vi "Main.vi"() -> ()   [LabVIEW 2021]
uses:
  TypeDef/StateMachine.ctl
  TypeDef/KeyDown.ctl
  GlobalVariables/Global_KeyDown.vi
  GlobalVariables/Board_Colors.vi
panel:
  in  "stop":bool
  out "Scoreboard":i32
  out "Level":u32[][](array[colorbox])
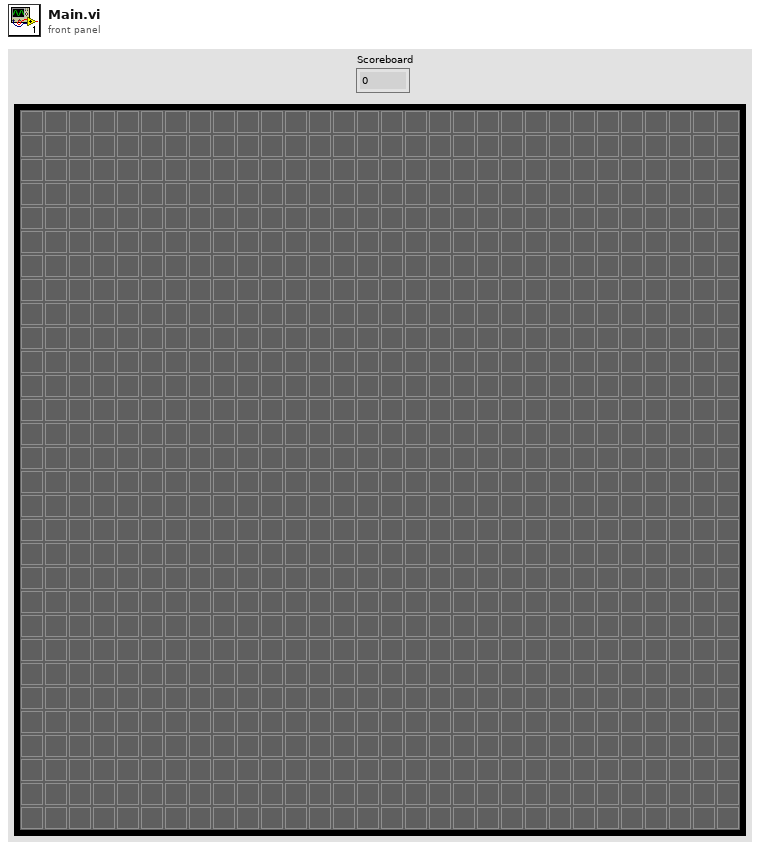
[diagram p1: front panel]
types:
  T1 = typedef "KeyDown.ctl" = enum16{"Up", "Down", "Left", "Right"}
  T2 = typedef "StateMachine.ctl" = enum16{"Init", "Game Logic", "Snake Growth", "Move", "Wait", "Food", "Update", "Game over"}
  T3 = typedef "eventvkey.ctl" = enum16{"ASCII", "Enter", "Return", "Shift", "Ctrl", "Alt", "Cmd", "Opt", "Caps", "NumLock", "Clear", "Break", "Up", "Down", "Left", "Right", "Insert", "Delete", "Home", "End", "PageUp", "PageDown", "Escape", "Help", "Pause", "ScrollLock", "F1", "F2", "F3", "F4", "F5", "F6", "F7", "F8", "F9", "F10", "F11", "F12", "F13", "F14", "F15", "F16", "F17", "F18", "F19", "F20", "F21", "F22", "F23", "F24", "Play", "VolumeUp", "VolumeDown", "Mute", "Two Byte Char"}
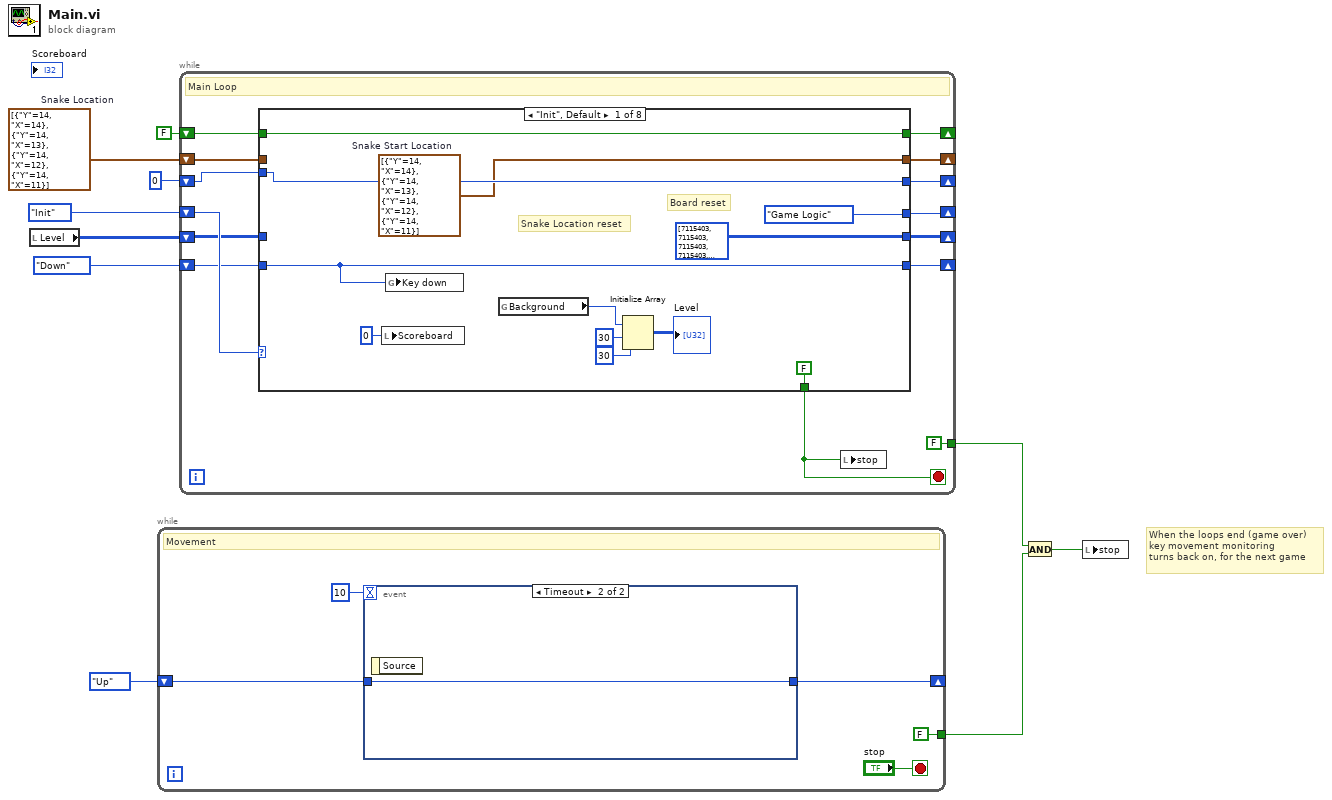
[diagram p0: block diagram]
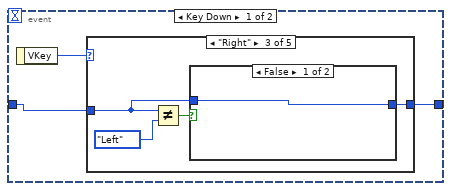
[diagram p2: hidden frame]
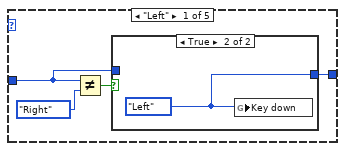
[diagram p3: hidden frame]
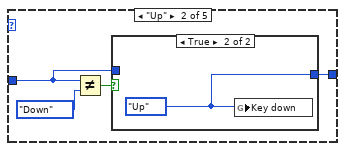
[diagram p5: hidden frame]
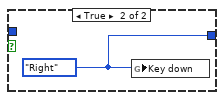
[diagram p7: hidden frame]
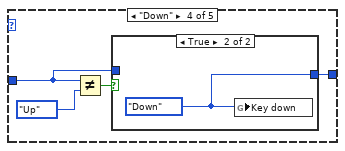
[diagram p8: hidden frame]
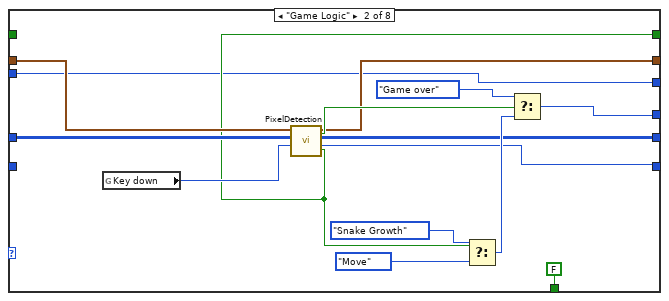
[diagram p11: hidden frame]
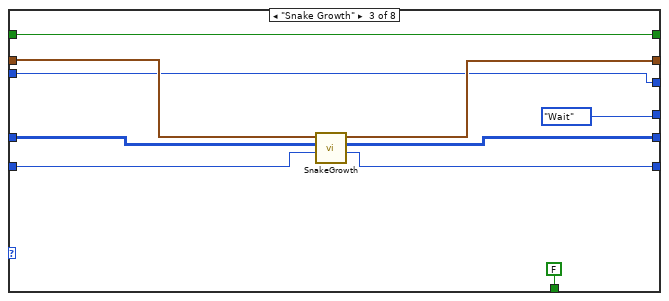
[diagram p12: hidden frame]
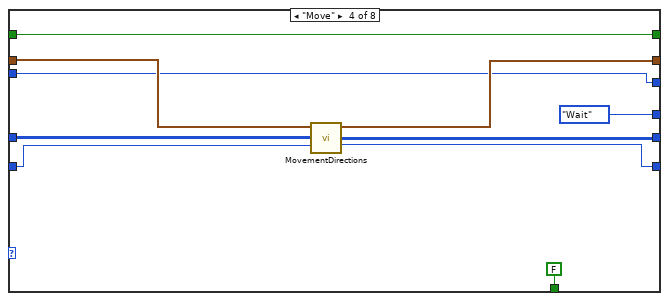
[diagram p13: hidden frame]
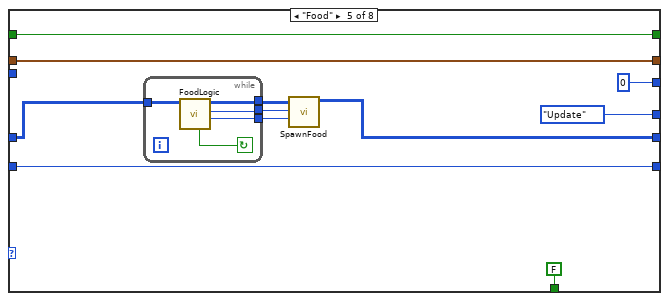
[diagram p14: hidden frame]
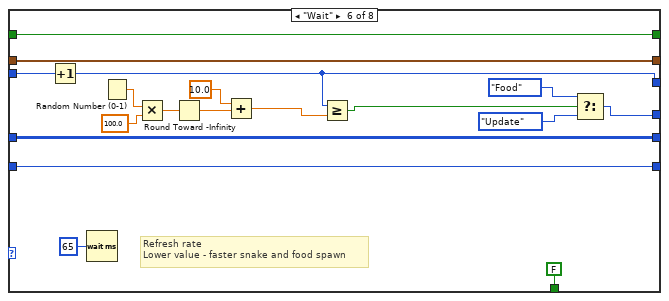
[diagram p15: hidden frame]
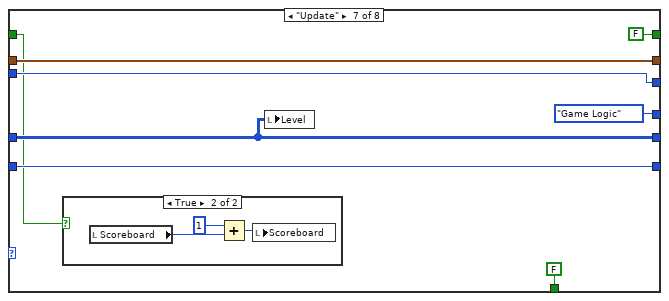
[diagram p16: hidden frame]
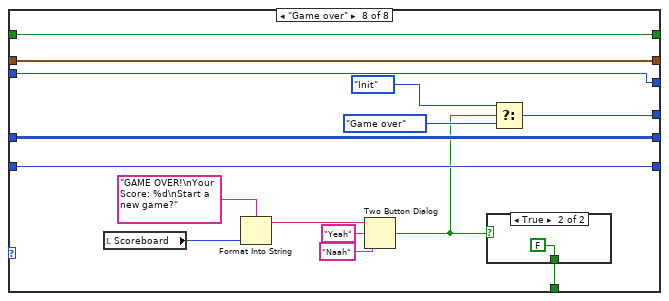
[diagram p18: hidden frame]
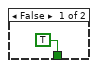
[diagram p19: hidden frame]
diagram:
  w9 = cluster{"Y":i32, "X":i32}[] [{"Y"=14, "X"=14}, {"Y"=14, "X"=13}, {"Y"=14, "X"=12}, {"Y"=14, "X"=11}]  # Snake Location
  # "When the loops end (game over)\nkey movement monitoring\nturns back on, for the next game"
  n1 = local read "Level"() -> (w8:u32[][])
  n2 = while {
    shift-right: [w13] -> _
    shift-left: KeyDown."Up" ("Key down") -> [w14]
    tunnel: [FALSE ("y")] -> w4
    stop <- "stop" stop-if-true
    # "Movement"
    n3 = event shown="[1] Timeout" {
      selector: _ -> [_ _]
      dyn-events: _ -> [_ _]
      timeout: 10 -> [_ _]
      tunnel: [w17 w44] -> w13
      tunnel: w14 -> [w16 w44]
      event Key Down {
        n4 = event-data() -> ("VKey"=w18:T3)  [unwired: 1 in]
        n5 = case shown="\"Right\"" w18 {
          tunnel: [w21 w27 w33 w39 w43] -> w17
          tunnel: w16 -> [w19 w25 w31 w37 w43]
          frame "Left" {
            n6 = Not Equal?(x=w19, y=KeyDown."Right" ("Key down")) -> (x != y?=w22:bool)
            n7 = case shown="True" w22 {
              tunnel: [w23 w24] -> w21
              tunnel: w19 -> [w23 _]
              frame False {
              }
              frame True {
                w24 = KeyDown."Left" ("Key down")
                n8 = global write "Global_KeyDown.vi" "Key down"(w24) -> ()
              }
            }
          }
          frame "Up" {
            n9 = Not Equal?(x=w25, y=KeyDown."Down" ("Key down")) -> (x != y?=w28:bool)
            n10 = case shown="True" w28 {
              tunnel: [w29 w30] -> w27
              tunnel: w25 -> [w29 _]
              frame False {
              }
              frame True {
                w30 = KeyDown."Up" ("Key down")
                n11 = global write "Global_KeyDown.vi" "Key down"(w30) -> ()
              }
            }
          }
          frame "Right" {
            n12 = Not Equal?(x=w31, y=KeyDown."Left" ("Key down")) -> (x != y?=w34:bool)
            n13 = case shown="False" w34 {
              tunnel: [w35 w36] -> w33
              tunnel: w31 -> [w35 _]
              frame False {
              }
              frame True {
                w36 = KeyDown."Right" ("Key down")
                n14 = global write "Global_KeyDown.vi" "Key down"(w36) -> ()
              }
            }
          }
          frame "Down" {
            n15 = Not Equal?(x=w37, y=KeyDown."Up" ("Key down")) -> (x != y?=w40:bool)
            n16 = case shown="True" w40 {
              tunnel: [w41 w42] -> w39
              tunnel: w37 -> [w41 _]
              frame False {
              }
              frame True {
                w42 = KeyDown."Down" ("Key down")
                n17 = global write "Global_KeyDown.vi" "Key down"(w42) -> ()
              }
            }
          }
          frame Default {
          }
        }
      }
      event Timeout {
        n18 = event-data() -> ()  [unwired: 1 in, 1 out]
      }
    }
  }
  n19 = while {
    shift-right: [w53] -> _
    shift-left: StateMachine."Init" -> [w58]
    shift-right: [w56] -> _
    shift-left: KeyDown."Down" ("Key down") -> [w57]
    shift-right: [w55] -> _
    shift-left: w9 -> [w54]
    shift-right: [w52] -> _
    shift-left: w8 -> [w51]
    tunnel: [FALSE] -> w5
    shift-right: [w49] -> _
    shift-left: 0 -> [w48]
    shift-right: [w47] -> _
    shift-left: FALSE -> [w46]
    stop <- w45 stop-if-true
    # "Main Loop"
    n20 = case shown="\"Init\", Default" w58 {
      tunnel: w57 -> [w69 _ w91 w101 w116 w137 w144 w165]
      tunnel: [w69 w79 w90 w100 w116 w137 w144 w165] -> w56
      tunnel: [w60 w77 w94 w104 w114 w139 w147 w164] -> w55
      tunnel: w54 -> [_ w83 w95 w105 w114 w139 w147 w164]
      tunnel: [StateMachine."Game Logic" w74 StateMachine."Wait" StateMachine."Wait" StateMachine."Update" w134 StateMachine."Game Logic" w155] -> w53
      tunnel: [u32[][] [[7115403, 7115403, 7115403, 7115403, 7115403, 7115403, 7115403, 7115403, 7115403, 7115403, 7115403, 7115403, 7115403, 7115403, 7115403, 7115403, 7115403, 7115403, 7115403, 7115403, 7115403, 7115403, 7115403, 7115403, 7115403, 7115403, 7115403, 7115403, 7115403, 7115403], [7115403, 7115403, 7115403, 7115403, 7115403, 7115403, 7115403, 7115403, 7115403, 7115403, 7115403, 7115403, 7115403, 7115403, 7115403, 7115403, 7115403, 7115403, 7115403, 7115403, 7115403, 7115403, 7115403, 7115403, 7115403, 7115403, 7115403, 7115403, 7115403, 7115403], [7115403, 7115403, 7115403, 7115403, 7115403, 7115403, 7115403, 7115403, 7115403, 7115403, 7115403, 7115403, 7115403, 7115403, 7115403, 7115403, 7115403, 7115403, 7115403, 7115403, 7115403, 7115403, 7115403, 7115403, 7115403, 7115403, 7115403, 7115403, 7115403, 7115403], [7115403, 7115403, 7115403, 7115403, 7115403, 7115403, 7115403, 7115403, 7115403, 7115403, 7115403, 7115403, 7115403, 7115403, 7115403, 7115403, 7115403, 7115403, 7115403, 7115403, 7115403, 7115403, 7115403, 7115403, 7115403, 7115403, 7115403, 7115403, 7115403, 7115403], [7115403, 7115403, 7115403, 7115403, 7115403, 7115403, 7115403, 7115403, 7115403, 7115403, 7115403, 7115403, 7115403, 7115403, 7115403, 7115403, 7115403, 7115403, 7115403, 7115403, 7115403, 7115403, 7115403, 7115403, 7115403, 7115403, 7115403, 7115403, 7115403, 7115403], [7115403, 7115403, 7115403, 7115403, 7115403, 7115403, 7115403, 7115403, 7115403, 7115403, 7115403, 7115403, 7115403, 7115403, 7115403, 7115403, 7115403, 7115403, 7115403, 7115403, 7115403, 7115403, 7115403, 7115403, 7115403, 7115403, 7115403, 7115403, 7115403, 7115403], [7115403, 7115403, 7115403, 7115403, 7115403, 7115403, 7115403, 7115403, 7115403, 7115403, 7115403, 7115403, 7115403, 7115403, 7115403, 7115403, 7115403, 7115403, 7115403, 7115403, 7115403, 7115403, 7115403, 7115403, 7115403, 7115403, 7115403, 7115403, 7115403, 7115403], [7115403, 7115403, 7115403, 7115403, 7115403, 7115403, 7115403, 7115403, 7115403, 7115403, 7115403, 7115403, 7115403, 7115403, 7115403, 7115403, 7115403, 7115403, 7115403, 7115403, 7115403, 7115403, 7115403, 7115403, 7115403, 7115403, 7115403, 7115403, 7115403, 7115403], [7115403, 7115403, 7115403, 7115403, 7115403, 7115403, 7115403, 7115403, 7115403, 7115403, 7115403, 7115403, 7115403, 7115403, 7115403, 7115403, 7115403, 7115403, 7115403, 7115403, 7115403, 7115403, 7115403, 7115403, 7115403, 7115403, 7115403, 7115403, 7115403, 7115403], [7115403, 7115403, 7115403, 7115403, 7115403, 7115403, 7115403, 7115403, 7115403, 7115403, 7115403, 7115403, 7115403, 7115403, 7115403, 7115403, 7115403, 7115403, 7115403, 7115403, 7115403, 7115403, 7115403, 7115403, 7115403, 7115403, 7115403, 7115403, 7115403, 7115403], [7115403, 7115403, 7115403, 7115403, 7115403, 7115403, 7115403, 7115403, 7115403, 7115403, 7115403, 7115403, 7115403, 7115403, 7115403, 7115403, 7115403, 7115403, 7115403, 7115403, 7115403, 7115403, 7115403, 7115403, 7115403, 7115403, 7115403, 7115403, 7115403, 7115403], [7115403, 7115403, 7115403, 7115403, 7115403, 7115403, 7115403, 7115403, 7115403, 7115403, 7115403, 7115403, 7115403, 7115403, 7115403, 7115403, 7115403, 7115403, 7115403, 7115403, 7115403, 7115403, 7115403, 7115403, 7115403, 7115403, 7115403, 7115403, 7115403, 7115403], [7115403, 7115403, 7115403, 7115403, 7115403, 7115403, 7115403, 7115403, 7115403, 7115403, 7115403, 7115403, 7115403, 7115403, 7115403, 7115403, 7115403, 7115403, 7115403, 7115403, 7115403, 7115403, 7115403, 7115403, 7115403, 7115403, 7115403, 7115403, 7115403, 7115403], [7115403, 7115403, 7115403, 7115403, 7115403, 7115403, 7115403, 7115403, 7115403, 7115403, 7115403, 7115403, 7115403, 7115403, 7115403, 7115403, 7115403, 7115403, 7115403, 7115403, 7115403, 7115403, 7115403, 7115403, 7115403, 7115403, 7115403, 7115403, 7115403, 7115403], [7115403, 7115403, 7115403, 7115403, 7115403, 7115403, 7115403, 7115403, 7115403, 7115403, 7115403, 7115403, 7115403, 7115403, 7115403, 7115403, 7115403, 7115403, 7115403, 7115403, 7115403, 7115403, 7115403, 7115403, 7115403, 7115403, 7115403, 7115403, 7115403, 7115403], [7115403, 7115403, 7115403, 7115403, 7115403, 7115403, 7115403, 7115403, 7115403, 7115403, 7115403, 7115403, 7115403, 7115403, 7115403, 7115403, 7115403, 7115403, 7115403, 7115403, 7115403, 7115403, 7115403, 7115403, 7115403, 7115403, 7115403, 7115403, 7115403, 7115403], [7115403, 7115403, 7115403, 7115403, 7115403, 7115403, 7115403, 7115403, 7115403, 7115403, 7115403, 7115403, 7115403, 7115403, 7115403, 7115403, 7115403, 7115403, 7115403, 7115403, 7115403, 7115403, 7115403, 7115403, 7115403, 7115403, 7115403, 7115403, 7115403, 7115403], [7115403, 7115403, 7115403, 7115403, 7115403, 7115403, 7115403, 7115403, 7115403, 7115403, 7115403, 7115403, 7115403, 7115403, 7115403, 7115403, 7115403, 7115403, 7115403, 7115403, 7115403, 7115403, 7115403, 7115403, 7115403, 7115403, 7115403, 7115403, 7115403, 7115403], [7115403, 7115403, 7115403, 7115403, 7115403, 7115403, 7115403, 7115403, 7115403, 7115403, 7115403, 7115403, 7115403, 7115403, 7115403, 7115403, 7115403, 7115403, 7115403, 7115403, 7115403, 7115403, 7115403, 7115403, 7115403, 7115403, 7115403, 7115403, 7115403, 7115403], [7115403, 7115403, 7115403, 7115403, 7115403, 7115403, 7115403, 7115403, 7115403, 7115403, 7115403, 7115403, 7115403, 7115403, 7115403, 7115403, 7115403, 7115403, 7115403, 7115403, 7115403, 7115403, 7115403, 7115403, 7115403, 7115403, 7115403, 7115403, 7115403, 7115403], [7115403, 7115403, 7115403, 7115403, 7115403, 7115403, 7115403, 7115403, 7115403, 7115403, 7115403, 7115403, 7115403, 7115403, 7115403, 7115403, 7115403, 7115403, 7115403, 7115403, 7115403, 7115403, 7115403, 7115403, 7115403, 7115403, 7115403, 7115403, 7115403, 7115403], [7115403, 7115403, 7115403, 7115403, 7115403, 7115403, 7115403, 7115403, 7115403, 7115403, 7115403, 7115403, 7115403, 7115403, 7115403, 7115403, 7115403, 7115403, 7115403, 7115403, 7115403, 7115403, 7115403, 7115403, 7115403, 7115403, 7115403, 7115403, 7115403, 7115403], [7115403, 7115403, 7115403, 7115403, 7115403, 7115403, 7115403, 7115403, 7115403, 7115403, 7115403, 7115403, 7115403, 7115403, 7115403, 7115403, 7115403, 7115403, 7115403, 7115403, 7115403, 7115403, 7115403, 7115403, 7115403, 7115403, 7115403, 7115403, 7115403, 7115403], [7115403, 7115403, 7115403, 7115403, 7115403, 7115403, 7115403, 7115403, 7115403, 7115403, 7115403, 7115403, 7115403, 7115403, 7115403, 7115403, 7115403, 7115403, 7115403, 7115403, 7115403, 7115403, 7115403, 7115403, 7115403, 7115403, 7115403, 7115403, 7115403, 7115403], [7115403, 7115403, 7115403, 7115403, 7115403, 7115403, 7115403, 7115403, 7115403, 7115403, 7115403, 7115403, 7115403, 7115403, 7115403, 7115403, 7115403, 7115403, 7115403, 7115403, 7115403, 7115403, 7115403, 7115403, 7115403, 7115403, 7115403, 7115403, 7115403, 7115403], [7115403, 7115403, 7115403, 7115403, 7115403, 7115403, 7115403, 7115403, 7115403, 7115403, 7115403, 7115403, 7115403, 7115403, 7115403, 7115403, 7115403, 7115403, 7115403, 7115403, 7115403, 7115403, 7115403, 7115403, 7115403, 7115403, 7115403, 7115403, 7115403, 7115403], [7115403, 7115403, 7115403, 7115403, 7115403, 7115403, 7115403, 7115403, 7115403, 7115403, 7115403, 7115403, 7115403, 7115403, 7115403, 7115403, 7115403, 7115403, 7115403, 7115403, 7115403, 7115403, 7115403, 7115403, 7115403, 7115403, 7115403, 7115403, 7115403, 7115403], [7115403, 7115403, 7115403, 7115403, 7115403, 7115403, 7115403, 7115403, 7115403, 7115403, 7115403, 7115403, 7115403, 7115403, 7115403, 7115403, 7115403, 7115403, 7115403, 7115403, 7115403, 7115403, 7115403, 7115403, 7115403, 7115403, 7115403, 7115403, 7115403, 7115403], [7115403, 7115403, 7115403, 7115403, 7115403, 7115403, 7115403, 7115403, 7115403, 7115403, 7115403, 7115403, 7115403, 7115403, 7115403, 7115403, 7115403, 7115403, 7115403, 7115403, 7115403, 7115403, 7115403, 7115403, 7115403, 7115403, 7115403, 7115403, 7115403, 7115403], [7115403, 7115403, 7115403, 7115403, 7115403, 7115403, 7115403, 7115403, 7115403, 7115403, 7115403, 7115403, 7115403, 7115403, 7115403, 7115403, 7115403, 7115403, 7115403, 7115403, 7115403, 7115403, 7115403, 7115403, 7115403, 7115403, 7115403, 7115403, 7115403, 7115403]] ("Level") w78 w92 w102 w113 w138 w146 w163] -> w52
      tunnel: w51 -> [_ w84 w93 w103 w112 w138 w146 w163]
      tunnel: [w67 w72 w88 w98 0 w124 w142 w162] -> w49
      tunnel: w48 -> [w67 w72 w88 w98 _ w125 w142 w162]
      tunnel: [w66 w73 w87 w97 w107 w123 FALSE w161] -> w47
      tunnel: w46 -> [w66 _ w87 w97 w107 w123 w141 w161]
      tunnel: [FALSE FALSE FALSE FALSE FALSE FALSE FALSE w153] -> w45
      frame "Init", Default {
        w60 = cluster{"Y":i32, "X":i32}[] [{"Y"=14, "X"=14}, {"Y"=14, "X"=13}, {"Y"=14, "X"=12}, {"Y"=14, "X"=11}]  # Snake Start Location
        # "Snake Location reset"
        # "Board reset"
        n21 = local write "Scoreboard"(0 ("Scoreboard")) -> ()
        n22 = global write "Global_KeyDown.vi" "Key down"(w69) -> ()
        n23 = global read "Board_Colors.vi" "Background"() -> (w64:u32)
        n24 = Initialize Array(w64, 30 ("dimension size"), 30 ("dimension size")) -> (→"Level":u32[][])
      }
      frame "Game Logic" {
        n25 = global read "Global_KeyDown.vi" "Key down"() -> (w85:T1)
        n26 = call "PixelDetection.vi"("Key input"=w85, "Level input"=w84, "Location input"=w83) -> ("Key output"=w79:T1, "Level output"=w78:u32[][], "Location output"=w77:cluster{"Y":i32, "X":i32}[], "Food eaten?"=w73:bool, "Game Over?"=w82:bool)  [unwired: 4 in]
        n27 = Select(t=StateMachine."Snake Growth", s=w73, f=StateMachine."Move") -> (s? t:f=w81:T2)
        n28 = Select(t=StateMachine."Game over", s=w82, f=w81) -> (s? t:f=w74:T2)
      }
      frame "Snake Growth" {
        n29 = call "SnakeGrowth.vi"("Key input"=w91, "Level input"=w93, "Location input"=w95) -> ("Key output"=w90:T1, "Level output"=w92:u32[][], "Location output"=w94:cluster{"Y":i32, "X":i32}[])  [unwired: 6 in]
      }
      frame "Move" {
        n30 = call "MovementDirections.vi"("Key input"=w101, "Level input"=w103, "Location input"=w105) -> ("Key output"=w100:T1, "Level output"=w102:u32[][], "Location output"=w104:cluster{"Y":i32, "X":i32}[])  [unwired: 6 in]
      }
      frame "Food" {
        n31 = while {
          tunnel: w112 -> [w120]
          tunnel: [w119] -> w111
          tunnel: [w118] -> w110
          tunnel: [w117] -> w109
          stop <- w121 continue-if-true
          n32 = call "FoodLogic.vi"("Level input"=w120) -> ("X Position"=w119:i32, "Y Position"=w118:i32, "Level output"=w117:u32[][], "Pixel Occupied?"=w121:bool)  [unwired: 7 in]
        }
        n33 = call "SpawnFood.vi"("X Position"=w111, "Y Position"=w110, "Level input"=w109) -> ("Level output"=w113:u32[][])  [unwired: 8 in]
      }
      frame "Wait" {
        # "Refresh rate\nLower value - faster snake and food spawn"
        n34 = Increment(x=w125) -> (x+1=w124:i32)
        n35 = Wait (ms)(milliseconds to wait=u32 65) -> ()  [unwired: 1 out]
        n36 = Random Number (0-1)() -> (number: 0 to 1=w131:dbl)
        n37 = Multiply(x=w131, y=100.0) -> (x*y=w130:dbl)
        n38 = Round Toward -Infinity(1:w130) -> (0:w128:dbl)
        n39 = Add(x=10.0, y=w128) -> (x+y=w127:dbl)
        n40 = Greater Or Equal?(x=w124, y=w127) -> (x >= y?=w126:bool)
        n41 = Select(t=StateMachine."Food", s=w126, f=StateMachine."Update") -> (s? t:f=w134:T2)
      }
      frame "Update" {
        n42 = case shown="True" w141 {
          frame False {
          }
          frame True {
            n43 = local read "Scoreboard"() -> (w150:i32)
            n44 = Add(x=1, y=w150) -> (x+y=w148:i32)
            n45 = local write "Scoreboard"(w148) -> ()
          }
        }
        n46 = local write "Level"(w146) -> ()
      }
      frame "Game over" {
        n47 = local read "Scoreboard"() -> (w160:i32)
        n48 = Format Into String(format string="GAME OVER!\nYour Score: %d\nStart a new game?", w160) -> (resulting string=w159:string)  [unwired: 2 in, 1 out]
        n49 = Two Button Dialog(message=w159, 1:"Naah" ("F button name (\"Cancel\")"), 2:"Yeah" ("T button name (\"OK\")")) -> (T button?=w154:bool)
        n50 = case shown="True" w154 {
          tunnel: [TRUE FALSE] -> w153
          frame False {
          }
          frame True {
          }
        }
        n51 = Select(t=StateMachine."Init", s=w154, f=StateMachine."Game over") -> (s? t:f=w155:T2)
      }
    }
    n52 = local write "stop"(w45) -> ()
  }
  n53 = And(x=w5, y=w4) -> (x .and. y?=w3:bool)
  n54 = local write "stop"(w3) -> ()
